vi "TCP-Find Next Available Port.vi"(5 "start":u16=4900) -> (6 "port":u16, 15 "error out":errorcluster)   [LabVIEW 2020]
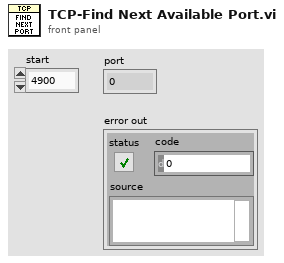
[diagram p1: front panel]
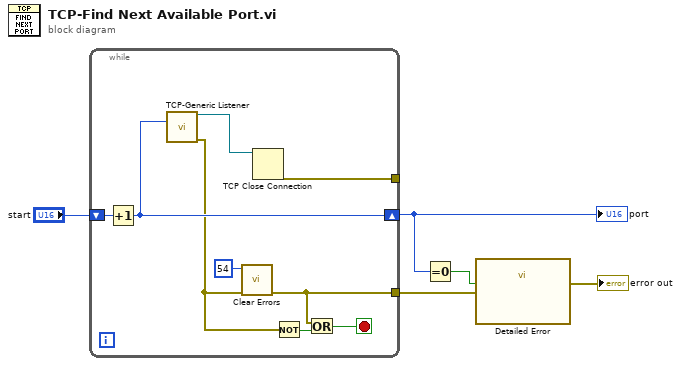
[diagram p0: block diagram]
diagram:
  n1 = while {
    tunnel: [w9] -> w3
    tunnel: [w13] -> _
    shift-right: [w8] -> w4
    shift-left: "start" -> [w14]
    stop <- w10 stop-if-true
    n2 = Increment(x=w14) -> (x+1=w8:u16)
    n3 = call "TCP-Generic Listener.vi"("port"=w8) -> ("connection ID"=w6:refnum<k5>, "error out"=w7:errorcluster)  [unwired: 12 in, 1 out]
    n4 = call <vilib>:"Clear Errors.vi"("error in (no error)"=w7, "specific error code to clear (0: all)"=54) -> ("error out"=w9:errorcluster)  [unwired: 4 in, 1 out]
    n5 = TCP Close Connection(connection ID=w6) -> (error out=w13:errorcluster)  [unwired: 2 in, 1 out]
    n6 = Not(x=w7) -> (.not. x?=w11:bool)
    n7 = Or(x=w9, y=w11) -> (x .or. y?=w10:bool)
  }
  "port" <- w4
  n8 = Equal To 0?(x=w4) -> (x = 0?=w2:bool)
  n9 = call "Detailed Error"("Error?"=w2, "Primary"=w3) -> ("detailed error"=→"error out":errorcluster)  [unwired: 13 in]
